vi "Send Ping Packet.vi"(0 "Socket To Use":u32 format="%04x", 5 "Resolved Host IP":u32 format="%x", 9 "Packet to Send":u8[](array[numeric]) format="%02x", 11 "Error In":errorcluster) -> (3 "TxTimeStamp":u32, 4 "Socket To Use Out":u32 format="%04x", 6 "Bytes Sent":i32, 8 "Resolved Host IP Out":u32 format="%x", 15 "Error Out":errorcluster)   [LabVIEW 2018]
uses:
  ws2_32.dll
panel:
  out "(sockaddr*)dest":u8[](array[numeric]) format="%02x"
  # "Send an ICMP echo (\"ping\") packet to host dest by way of sd with\npacket_size bytes.  packet_size is the total size of the ping packet\nto send, including the ICMP header and the payload area; it is not\nchecked for sanity, so make sure that it's at least \nsizeof(ICMPHeader) bytes, and that send_buf points to at least\npacket_size bytes.  Returns < 0 for failure"
  # "Type"
  # "Code"
  # "Checksum"
  # "Process ID"
  # "Sequence"
  # "Timestamp"
  # "Filler"
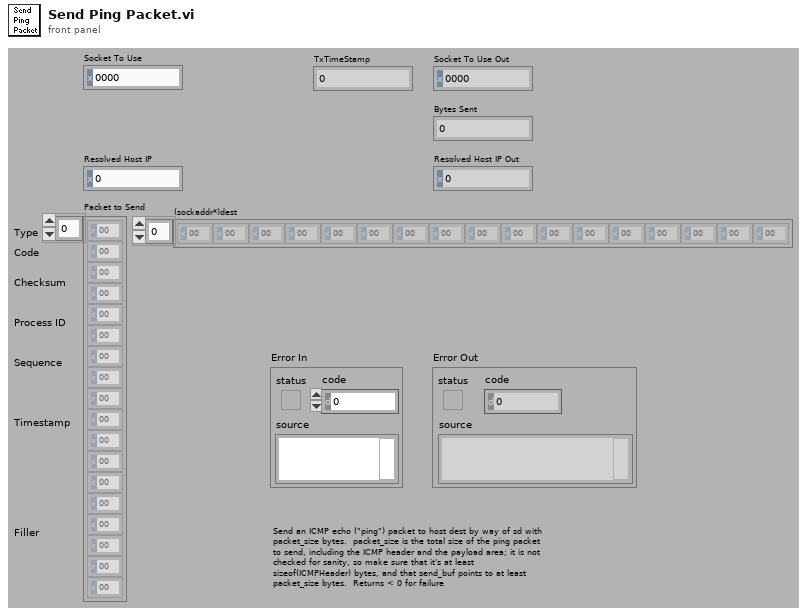
[diagram p1: front panel]
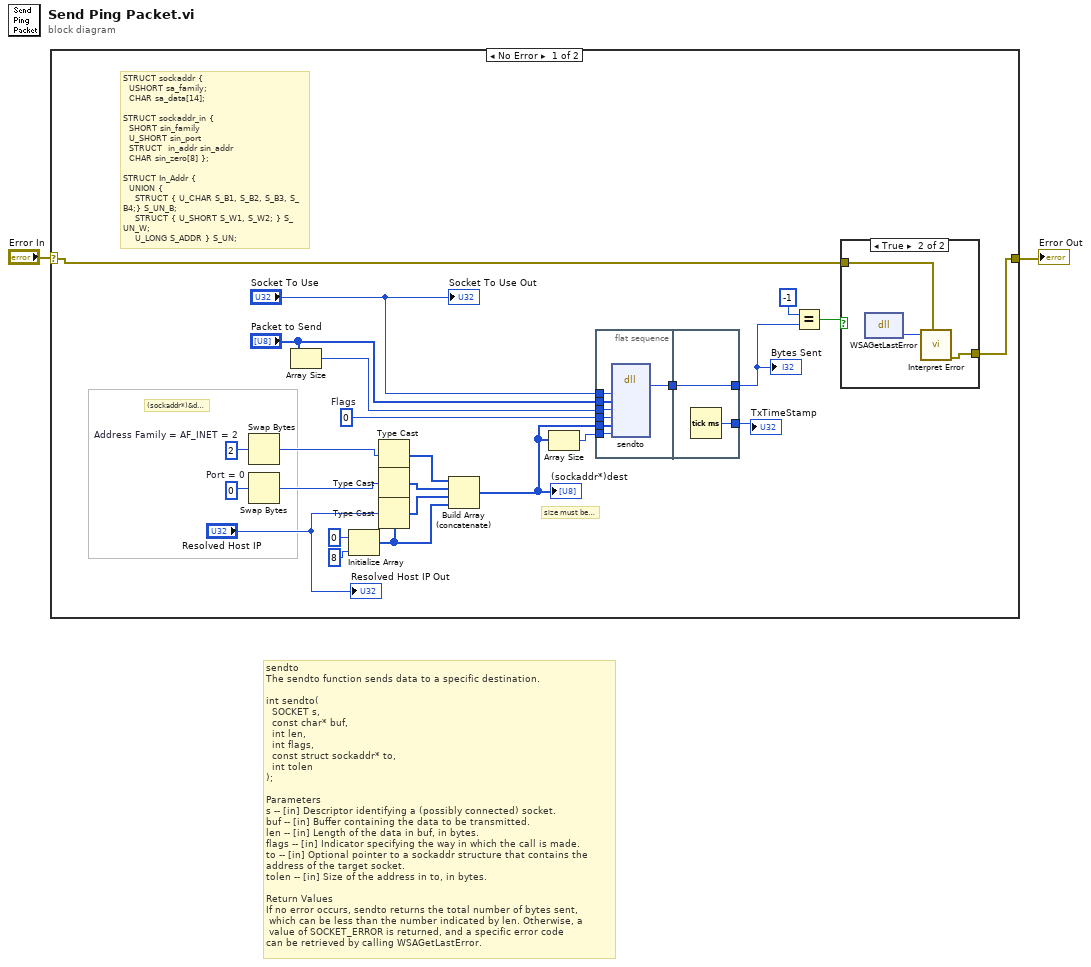
[diagram p0: block diagram]
diagram:
  # "sendto\nThe sendto function sends data to a specific destination.\n\nint sendto(\n  SOCKET s,\n  const char* buf,\n  int len,\n  int flags,\n  const struct sockaddr* to,\n  int tolen\n);\n\nParameters\ns -- [in] Descriptor identifying a (possibly connected) socket. \nbuf -- [in] Buffer containing the data to be transmitted. \nlen -- [in] Length of the data in buf, in bytes. \nflags -- [in] Indicator specifying the way in which the call is made. \nto -- [in] Optional pointer to a sockaddr structure that contains the address of the target socket. \ntolen -- [in] Size of the address in to, in bytes. \n\nReturn Values\nIf no error occurs, sendto returns the total number of bytes sent,\n which can be less than the number indicated by len. Otherwise, a\n value of SOCKET_ERROR is returned, and a specific error code \ncan be retrieved by calling WSAGetLastError."
  n1 = case shown="No Error" "Error In" {
    selector: "Error In" -> [w24 w40]
    tunnel: [w23 w40] -> w1
    frame No Error {
      w17 = u16 0  # Port = 0
      w19 = u16 2  # Address Family = AF_INET = 2
      w20 = 0  # Flags
      # "size must be 16"
      # "STRUCT sockaddr {\n  USHORT sa_family;\n  CHAR sa_data[14];\n\nSTRUCT sockaddr_in {\n  SHORT sin_family\n  U_SHORT sin_port\n  STRUCT  in_addr sin_addr\n  CHAR sin_zero[8] };\n\nSTRUCT In_Addr {\n  UNION {\n    STRUCT { U_CHAR S_B1, S_B2, S_B3, S_B4;} S_UN_B;\n    STRUCT { U_SHORT S_W1, S_W2; } S_UN_W;\n    U_LONG S_ADDR } S_UN;"
      # "(sockaddr*)&dest"
      n2 = Swap Bytes(anything=w19) -> (byte swapped=w6:u16)
      n3 = Swap Bytes(anything=w17) -> (byte swapped=w10:u16)
      n4 = Array Size(array="Packet to Send") -> (size(s)=w21:i32)
      n5 = Initialize Array(u8 0, u8 8) -> (w8:u8[])
      n6 = Type Cast(type=w8, x=w6) -> (*(type *) &x=w7:u8[])
      n7 = Type Cast(type=w8, x=w10) -> (*(type *) &x=w9:u8[])
      n8 = Type Cast(type=w8, x="Resolved Host IP") -> (*(type *) &x=w11:u8[])
      n9 = Build Array (concatenate)(w7, w9, w11, w8) -> (w18:u8[])
      "(sockaddr*)dest" <- w18
      n10 = Array Size(array=w18) -> (size(s)=w13:i32)
      n11 = flat-sequence {
        tunnel: "Packet to Send" -> [w32]
        tunnel: w21 -> [w31]
        tunnel: w20 -> [w30]
        tunnel: w18 -> [w29]
        tunnel: "Socket To Use" -> [w28]
        tunnel: w13 -> [w27]
        tunnel: [w33] -> w4
        tunnel: [w35] -> w26
        tunnel: w4 -> [w35]
        tunnel: [w34] -> w3
        frame #0 {
          n12 = dll-call lib="ws2_32.dll" fn="sendto" label="SendTo"("Socket"=w28, "Packet to Send"=w32, "Packet Length"=w31, "Flags"=w30, "Destination"=w29, "Dest Addr Len"=w27) -> ("Bytes Sent"=w33:i32)  [unwired: 9 in, 2 out]
        }
        frame #1 {
          n13 = Tick Count (ms)() -> (millisecond timer value=w34:u32)
        }
      }
      n14 = Equal?(x=-1, y=w26) -> (x = y?=w25:bool)
      n15 = case shown="True" w25 {
        tunnel: w24 -> [w36 w39]
        tunnel: [w36 w37] -> w23
        frame False {
        }
        frame True {
          n16 = dll-call lib="ws2_32.dll" fn="WSAGetLastError"() -> (w38:i32)  [unwired: 3 in, 2 out]
          n17 = call "Interpret Error.vi"("Error In"=w39, "Code"=w38) -> ("Error Out"=w37:errorcluster)  [unwired: 9 in]
        }
      }
      "Bytes Sent" <- w26
      "Resolved Host IP Out" <- "Resolved Host IP"
      "Socket To Use Out" <- "Socket To Use"
      "TxTimeStamp" <- w3
    }
    frame Error {
    }
  }
  "Error Out" <- w1
